vi "Read NumberOfRobots.vi"(8 "error in (no error)":errorcluster, 11 "5RobotsNormalGamePlay in":refnum<class "5RobotsNormalGamePlay.lvclass">) -> (0 "error out":errorcluster, 2 "NumberOfRobots":dbl=5.0, 3 "5RobotsNormalGamePlay out":refnum<class "5RobotsNormalGamePlay.lvclass">)   [LabVIEW 2023, in "5RobotsNormalGamePlay.lvclass"]
uses:
  5RobotsNormalGamePlay.lvclass
  5RobotsNormalGamePlay.lvclass/5RobotsNormalGamePlay.ctl
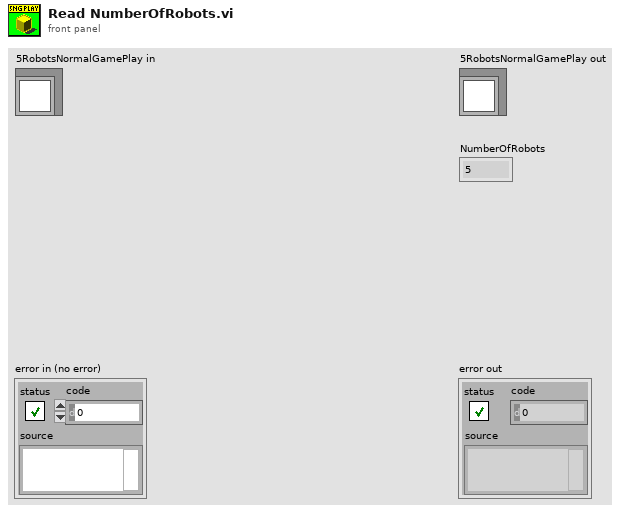
[diagram p1: front panel]
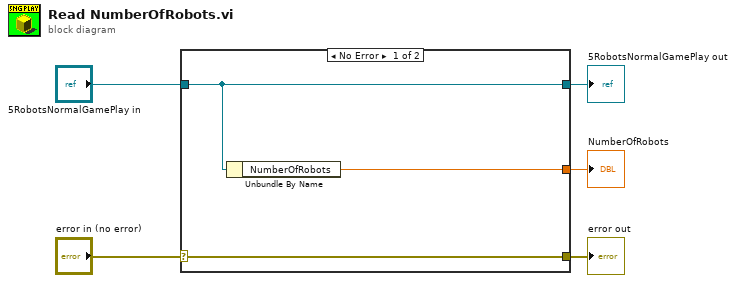
[diagram p0: block diagram]
diagram:
  n1 = case shown="No Error" "error in (no error)" {
    selector: "error in (no error)" -> [w8 w9]
    tunnel: [w8 w9] -> w4
    tunnel: [w7 w10] -> w2
    tunnel: "5RobotsNormalGamePlay in" -> [w7 w10]
    tunnel: [w6 _] -> w1
    frame No Error {
      n2 = Unbundle By Name(w7) -> ("NumberOfRobots"=w6:dbl)
    }
    frame Error {
    }
  }
  "error out" <- w4
  "5RobotsNormalGamePlay out" <- w2
  "NumberOfRobots" <- w1
